vi "Laser Control.vi"() -> ()   [LabVIEW 2012]
uses:
  <vilib>/rvi/interface/nirviOpenFPGA/nirviOpenFPGA.xnode
  FPGA Bitfiles/CRDSPAS_RIO0_FPGAIO_8FC4ABDC.lvbitx
  <vilib>/userdefined/High Color/nirio_resource_hc.ctl
  Utilities/FPGA/Controls/FPGA Signal.ctl
  <vilib>/rvi/interface/nirviReadWriteControl/nirviReadWriteControl.xnode
  <vilib>/rvi/interface/nirviCloseFPGA/nirviCloseFPGA.xnode
  <vilib>/FPGAPlugInAG/PXI-7841R/niLvFpga_Close_PXI-7841R.vi
  <vilib>/FPGAPlugInAG/PXI-7841R/niLvFpga_Open_PXI-7841R.vi
  NiFpgaLv.dll
  <vilib>/Utility/error.llb/Error Cluster From Error Code.vi
  <vilib>/rvi/errors/niLvFpgaAdjustHostInterfaceError.vi
panel:
  in  "Boolean":bool
  out "error out 3":errorcluster
  out "error out 2":errorcluster
  out "error out":errorcluster
  in  "WaveType":T1
  in  "f0":T2
  in  "FPGA Output":T3
  in  "stop":bool
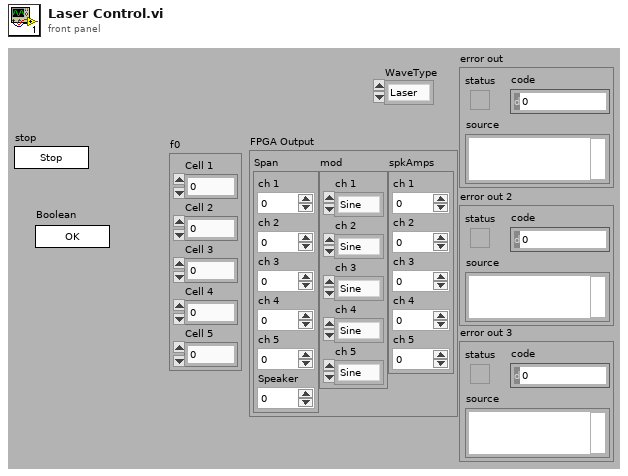
[diagram p1: front panel]
types:
  T1 = typedef "FPGA Signal.ctl" = enum16{"Laser", "None", "Speaker"}
  T2 = cluster{"Cell 1":sgl, "Cell 2":sgl, "Cell 3":sgl, "Cell 4":sgl, "Cell 5":sgl}
  T3 = cluster{"Span":cluster{"ch 1":sgl, "ch 2":sgl, "ch 3":sgl, "ch 4":sgl, "ch 5":sgl, "Speaker":sgl}, "mod":cluster{"ch 1":enum8{"Sine", "Square"}, "ch 2":enum8{"Sine", "Square"}, "ch 3":enum8{"Sine", "Square"}, "ch 4":enum8{"Sine", "Square"}, "ch 5":enum8{"Sine", "Square"}}, "spkAmps":cluster{"ch 1":sgl, "ch 2":sgl, "ch 3":sgl, "ch 4":sgl, "ch 5":sgl}}
  T4 = typedef "nirio_resource_hc.ctl" = tag
  T5 = cluster{"ch 1":sgl, "ch 2":sgl, "ch 3":sgl, "ch 4":sgl, "ch 5":sgl, "Speaker":sgl}
  T6 = cluster{"ch 1":enum8{"Sine", "Square"}, "ch 2":enum8{"Sine", "Square"}, "ch 3":enum8{"Sine", "Square"}, "ch 4":enum8{"Sine", "Square"}, "ch 5":enum8{"Sine", "Square"}}
  T7 = typedef "FxdPt Props.ctl" = cluster{"f0":fxp<+,32,0>, "Scale":fxp<+,14,1>, "Offset":i16, "Mod":T8}
  T8 = typedef "Laser Modulation.ctl" = enum8{"Sine", "Square"}
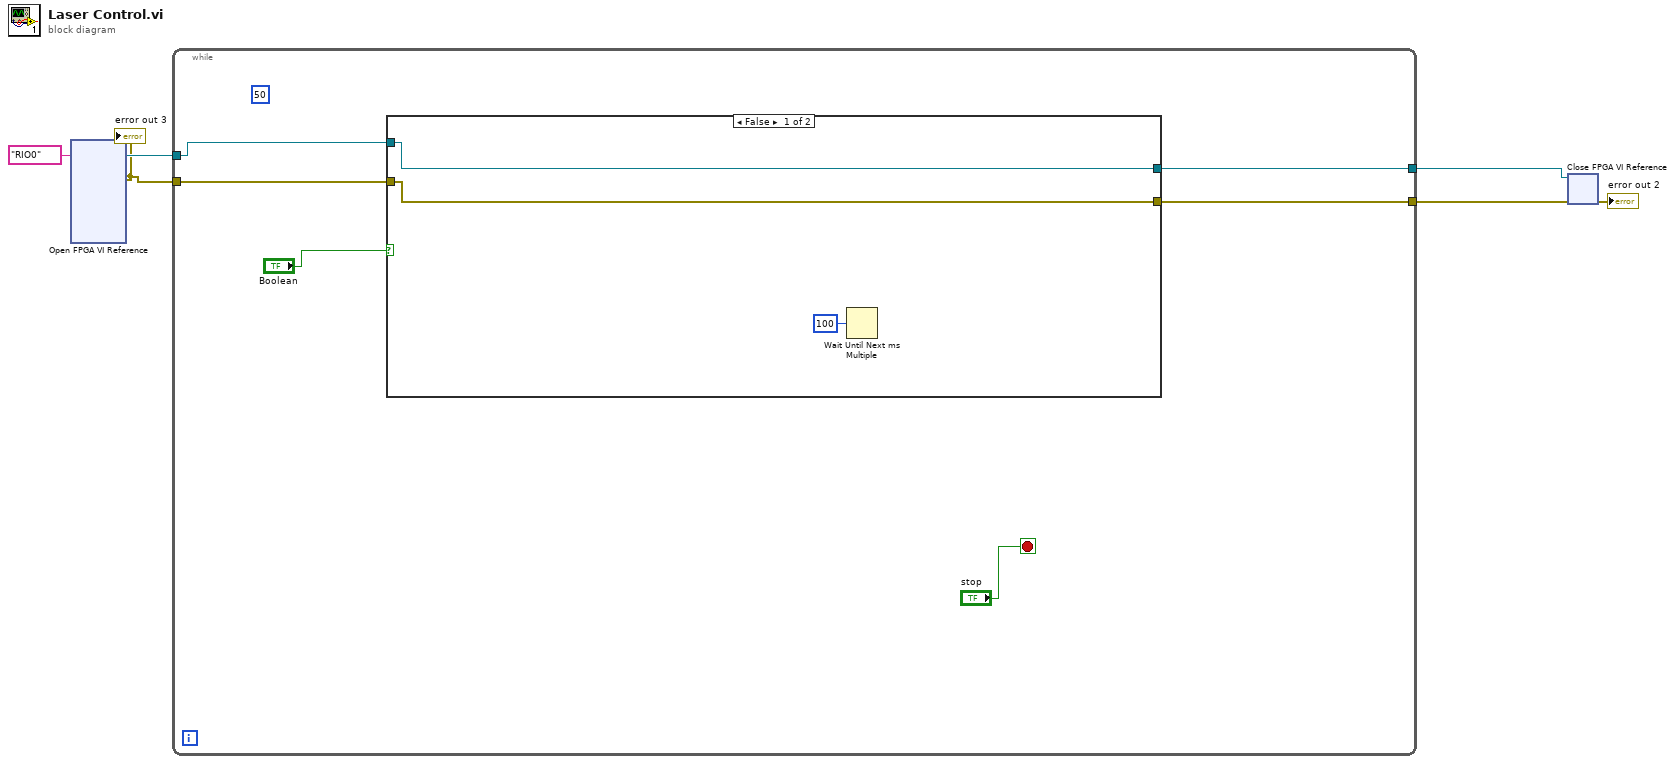
[diagram p0: block diagram]
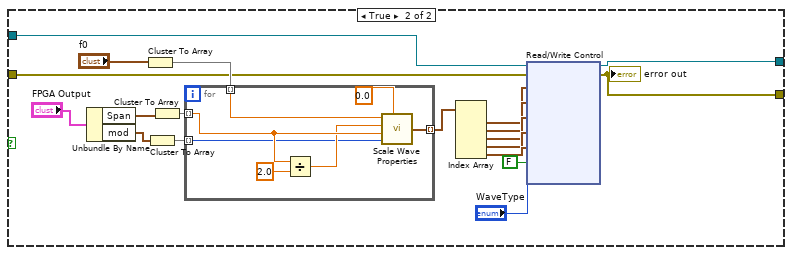
[diagram p2: hidden frame]
diagram:
  n1 = xnode "Open FPGA VI Reference"("resource name"=T4 "RIO0") -> ("FPGA VI Reference Out"=w6:refnum<k20>, "error out"=w4:errorcluster)  [unwired: 1 in]
  "error out 3" <- w4
  n2 = while {
    tunnel: w6 -> [w11]
    tunnel: w4 -> [w10]
    tunnel: [w9] -> w2
    tunnel: [w8] -> w1
    stop <- "stop" stop-if-true
    (unwired) 50
    n3 = case shown="False" "Boolean" {
      tunnel: w11 -> [w15 w19]
      tunnel: w10 -> [w14 w18]
      tunnel: [w15 w17] -> w9
      tunnel: [w14 w16] -> w8
      frame False {
        n4 = Wait Until Next ms Multiple(millisecond multiple=u32 100) -> ()  [unwired: 1 out]
      }
      frame True {
        n5 = Unbundle By Name("FPGA Output") -> ("Span"=w21:T5, "mod"=w23:T6)
        n6 = Cluster To Array(cluster="f0") -> (array=w26:sgl[])
        n7 = Cluster To Array(cluster=w23) -> (array=w24:enum8{"Sine", "Square"}[])
        n8 = Cluster To Array(cluster=w21) -> (array=w22:sgl[])
        n9 = for {
          tunnel: [w41] -> w27 mode=indexing
          tunnel: w22 -> [w38] mode=indexing
          tunnel: w24 -> [w35] mode=indexing
          tunnel: w26 -> [w40] mode=indexing
          n10 = Divide(x=w38, y=sgl 2.0) -> (x/y=w36:sgl)
          n11 = call "Scale Wave Properties.vi"("f0"=w40, "DCoffset"=w36, "Vspan"=w38, "Mod"=w35, 4:sgl 0.0 ("Amp")) -> ("FXP Props"=w41:T7)
        }
        n12 = Index Array(array=w27) -> (element #1=w28:T7, element #2=w29:T7, element #3=w30:T7, element #4=w31:T7, element #5=w32:T7)  [unwired: 5 in]
        n13 = xnode "Read/Write Control"("FPGA VI Reference In"=w19, "error in"=w18, "Cell 1"=w28, "Cell 2"=w29, "Cell 3"=w30, "Cell 4"=w31, "Cell 5"=w32, "Drive"=FALSE, "WaveType"="WaveType") -> ("FPGA VI Reference Out"=w17:refnum<k20>, "error out"=w16:errorcluster)
        "error out" <- w16
      }
    }
  }
  n14 = xnode "Close FPGA VI Reference"("FPGA VI Reference In"=w2, "error in"=w1) -> ("error out"=→"error out 2":errorcluster)
